vi "Generate Speaker Signal.vi"   [LabVIEW 2014]
doc: "The speaker signal is a chirp in the time domain and has the appearance of a tophat in the frequency domain. This signal generates an approximately constant voltage across a range of frequencies. Since the signal is symetric, the code will first cycle forward and then backward each second that the signal is generated. Half of the full speaker signal is stored in the memory labeled <b>Speaker Signal</b>.\n\nThe amplitude of the speaker signal is defied by the values <b>Voltage</b> and <b>Offset</b> stored in FPGA registers with the same name. The value <b>Voltage</b> is a fixed point number that ranges between 0 and 2 V, the limits of the speaker output. The value <b>Offset</b> allows the host to define an offset. The offset allows the card to produce a signal that does not traverse 0. The signal is expected to be AC coupled such that it fits the limits of the speaker specifications.\n\nThe speaker signal can be generated continuously . However, to prevent buzzing in the cavity, the host will have to disable the output via the Speaker Enable signal."
uses:
  <vilib>/rvi/FXPMathLib/FxpMul/XNode/nifxpmath_Multiplier.xnode
  <vilib>/rvi/FXPMathLib/FxpAdd/XNode/nifxpmath_Add.xnode
  <vilib>/eio/EIONode/EIONode.xnode
  <vilib>/rvi/DataTransferAndStorage/Container/XNode/niFpgaContainer.xnode
  <vilib>/rvi/Memory/Memory_Emulation/nirvimemoryEmulation.vi
  <vilib>/rvi/Memory/Memory_Emulation/nirvimemoryFastEmulation.vi
  <vilib>/rvi/DataTransferAndStorage/Register/Emulation/niFpgaRegisterEmulation.vi
  <vilib>/rvi/FXPMathLib/sim/FxpSim.dll
  <vilib>/rvi/eio/common/nirviEmuTemplateMethod_errors.vi
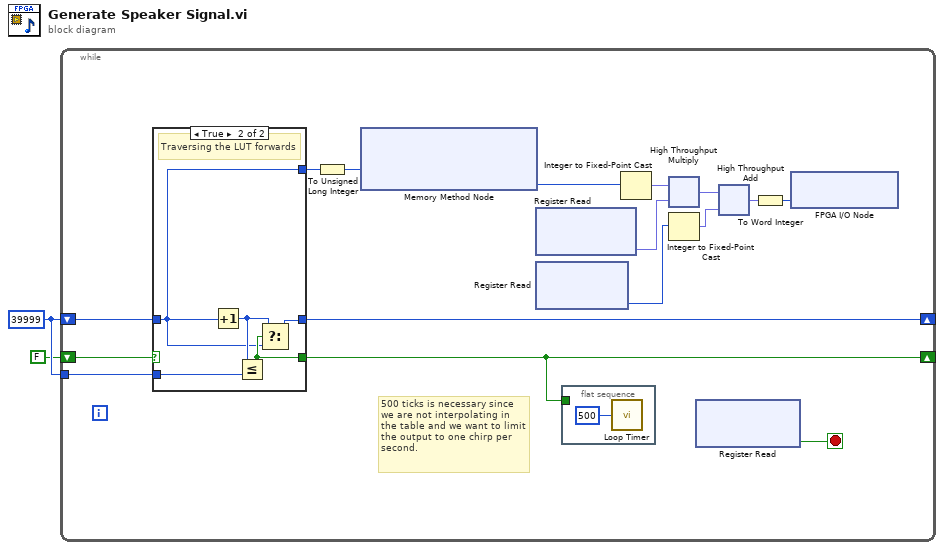
[diagram p0: block diagram]
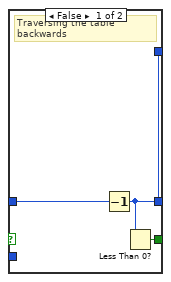
[diagram p2: hidden frame]
diagram:
  w2 = 39999
  n1 = while {
    shift-right: [w15] -> _
    shift-left: FALSE -> [w18]
    shift-right: [w16] -> _
    shift-left: w2 -> [w17]
    tunnel: w2 -> [w8]
    stop <- w5 stop-if-true
    # "500 ticks is necessary since we are not interpolating in the table and we want to limit the output to one chirp per second."
    n2 = case "Check where we are in the chirp" shown="True" w18 {
      tunnel: w17 -> [w20 w24]
      tunnel: [w22 w26] -> w15
      tunnel: [w20 w24] -> w7
      tunnel: [w21 w25] -> w16
      tunnel: w8 -> [_ w23]
      frame False {
        # "Traversing the table backwards"
        n3 = Decrement(x=w20) -> (x-1=w21:i32)
        n4 = Less Than 0?(x=w21) -> (x < 0?=w22:bool)
      }
      frame True {
        # "Traversing the LUT forwards"
        n5 = Increment(x=w24) -> (x+1=w27:i32)
        n6 = Less Or Equal?(x=w27, y=w23) -> (x <= y?=w26:bool)
        n7 = Select(t=w27, s=w26, f=w24) -> (s? t:f=w25:i32)
      }
    }
    n8 = To Unsigned Long Integer(number=w7) -> (unsigned 32bit integer=w6:u32)
    n9 = xnode ("Memory Method Node")("Address"=w6) -> ("Data"=w9:i16)  [unwired: 1 in, 1 out]
    n10 = xnode ("Register Read")() -> ("Data"=w3:fxp<+,32,0>)  [unwired: 1 in, 1 out]
    n11 = xnode ("Register Read")() -> ("Data"=w4:i16)  [unwired: 1 in, 1 out]
    n12 = flat-sequence {
      tunnel: w15 -> [_]
      frame #0 {
        n13 = call "Loop Timer"("Count(Ticks)"=u32 500) -> ()  [unwired: 1 out]
      }
    }
    n14 = Integer to Fixed-Point Cast(integer=w9) -> (fixed-point=w12:fxp<+/-,16,16>)  [unwired: 1 in]
    n15 = xnode ("High Throughput Multiply")("x"=w12, "y"=w3) -> ("x*y"=w14:fxp<+/-,48,16>)
    n16 = Integer to Fixed-Point Cast(integer=w4) -> (fixed-point=w13:fxp<+/-,16,16>)  [unwired: 1 in]
    n17 = xnode ("Register Read")() -> ("Data"=w5:bool)  [unwired: 1 in, 1 out]
    n18 = xnode ("High Throughput Add")("x"=w14, "y"=w13) -> ("x+y"=w10:fxp<+/-,16,16>)
    n19 = To Word Integer(number=w10) -> (16bit integer=w11:i16)
    n20 = xnode "FPGA I/O Node"("Speaker Out"=w11) -> ()  [unwired: 1 in, 1 out]
  }
